vi "Menu Item Selected.vi"(8 "error in (no error)":errorcluster, 10 "CtlRef":refnum<vi>, 11 "SwipeMenu in":refnum<class "SwipeMenu.lvclass">) -> (0 "error out":errorcluster)   [LabVIEW 2019, in "SwipeMenu.lvclass"]
uses:
  SwipeMenu.lvclass
  SwipeMenu.lvclass/SwipeMenu.ctl
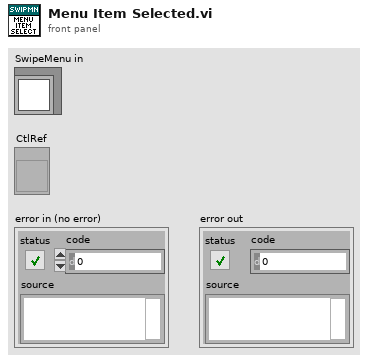
[diagram p1: front panel]
types:
  T1 = typedef "SwipeMenu.lvclass/State Data.ctl" = cluster{"State":enum16{"Idle", "Mouse Nav", "Slowdown", "Button Nav"}, "Timeout":i32, "Time":timestamp, "Position":i32, "Scroll Position":i16, "Rate":dbl, "Direction":enum16{"Left", "Right"}}
  T2 = enum16{"Idle", "Mouse Nav", "Slowdown", "Button Nav"}
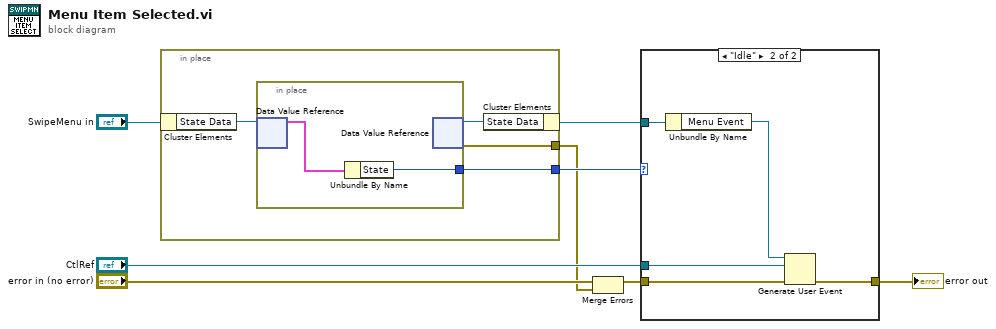
[diagram p0: block diagram]
diagram:
  n1 = in-place {
    in-place-border: [w10] -> w4
    in-place-border: [w9] -> w2
    n2 = in-place-cluster #1("SwipeMenu in") -> ("State Data"=w12:refnum<data-value>)
    n3 = in-place {
      in-place-border: [w13] -> w10
      n4 = in-place-dvr #2(w12) -> (w14:T1)  [unwired: 1 out]
      n5 = Unbundle By Name(w14) -> ("State"=w13:T2)
      n6 = in-place-dvr #2() -> (w11:refnum<data-value>, w9:errorcluster)  [unwired: 1 in]
    }
    n7 = in-place-cluster #1("State Data"=w11) -> (w5:refnum<class "SwipeMenu.lvclass">)
  }
  n8 = Merge Errors("error in (no error)", w2) -> (w1:errorcluster)
  n9 = case shown="\"Idle\"" w4 {
    tunnel: [w15 w20] -> w8
    tunnel: w1 -> [w15 w16]
    tunnel: "CtlRef" -> [_ w19]
    tunnel: w5 -> [_ w17]
    frame Default {
    }
    frame "Idle" {
      n10 = Unbundle By Name(w17) -> ("Menu Event"=w18:refnum<user-event>)
      n11 = Generate User Event(user event=w18, event data cluster=w19, error in=w16) -> (error out=w20:errorcluster)  [unwired: 1 in, 1 out]
    }
  }
  "error out" <- w8
